vi "Read.vi"(8 "error in (no error)":errorcluster, 11 "Concatenate_STR in":refnum<class "Concatenate_STR.lvclass">) -> (0 "error out":errorcluster, 2 "String":string, 3 "Concatenate_STR out":refnum<class "Concatenate_STR.lvclass">)   [LabVIEW 2021, in "Concatenate_STR.lvclass"]
uses:
  Concatenate_STR.lvclass
  Concatenate_STR.lvclass/Concatenate_STR.ctl
  Abs_Types/Value/Abs_Value.lvclass
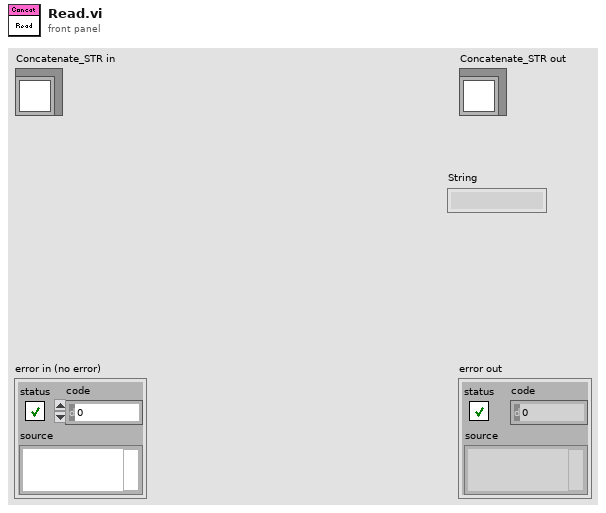
[diagram p1: front panel]
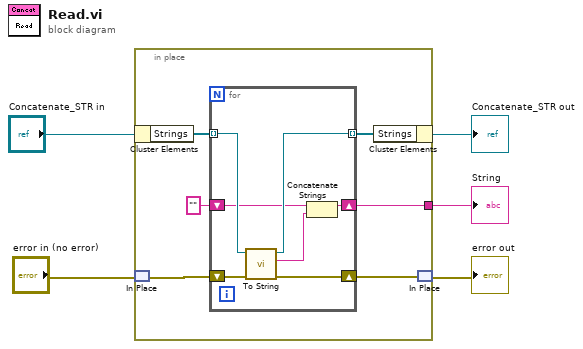
[diagram p0: block diagram]
diagram:
  n1 = in-place {
    in-place-border: [w7] -> w1
    n2 = in-place-cluster #1("Concatenate_STR in") -> ("Strings"=w10:refnum<class "Abs_Value.lvclass">[])
    n3 = in-place-match #2("error in (no error)") -> (w11:errorcluster)
    n4 = for {
      tunnel: w10 -> [w17] mode=indexing
      tunnel: [w16] -> w9 mode=indexing
      shift-right: [w15] -> w8
      shift-left: w11 -> [w18]
      shift-right: [w13] -> w7
      shift-left: "" -> [w12]
      n5 = call-dynamic "To String.vi"("error in (no error)"=w18, "Types in"=w17) -> ("error out"=w15:errorcluster, "String"=w14:string, "Types out"=w16:refnum<class "Abs_Value.lvclass">)  [unwired: 7 in]
      n6 = Concatenate Strings(w12, w14) -> (w13:string)
    }
    n7 = in-place-cluster #1("Strings"=w9) -> (→"Concatenate_STR out":refnum<class "Concatenate_STR.lvclass">)
    n8 = in-place-match #2(w8) -> (→"error out":errorcluster)
  }
  "String" <- w1
